vi "us_s_converter.vi"(4 "Time / us":dbl) -> (1 "Time / s":dbl)   [LabVIEW 2019]
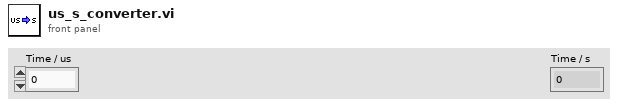
[diagram p1: front panel]
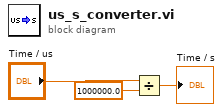
[diagram p0: block diagram]
diagram:
  n1 = Divide(x="Time / us", y=1000000.0) -> (x/y=→"Time / s":dbl)
